vi "UpdateElement(Single).vi"(7 "Qualified Name":string, 8 "error in (no error)":errorcluster, 9 "Value":string, 10 "Key":string, 11 "ConfigManager.Text in":refnum<class "ConfigManager.Text.lvclass">) -> (0 "error out":errorcluster, 3 "ConfigManager.Text out":refnum<class "ConfigManager.Text.lvclass">)   [LabVIEW 2013, in "CfgManager.Text.lvlib" / "ConfigManager.Text.lvclass"]
uses:
  ConfigManager.Text.lvclass
  ConfigManager.Text.lvclass/ConfigManager.Text.ctl
  Update -- cluster.ctl
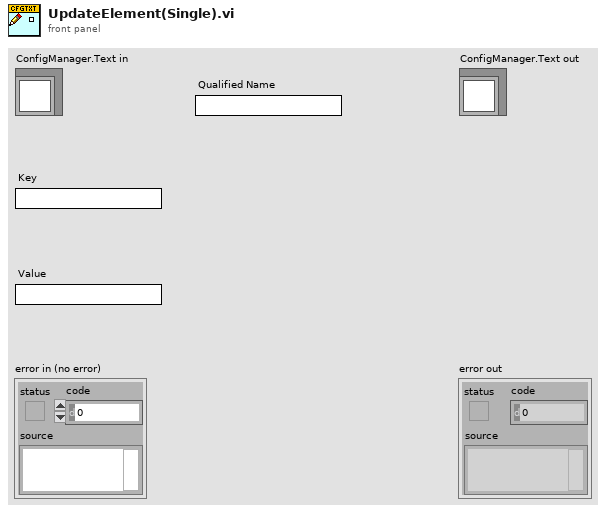
[diagram p1: front panel]
types:
  T1 = typedef "CfgManager.Text.lvlib/ConfigManager.Text.lvclass/Update -- cluster.ctl" = cluster{"Qualified Name":string[], "Keys":string[], "Values":string[]}
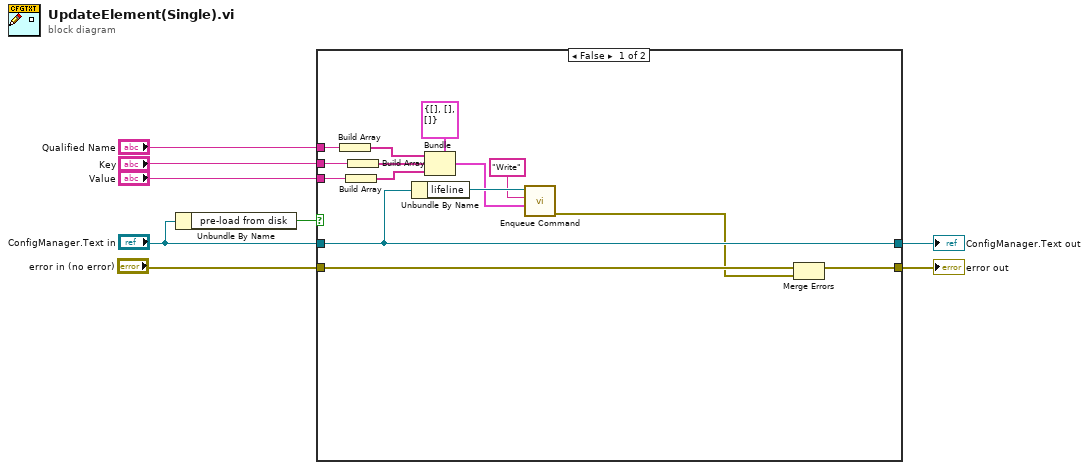
[diagram p0: block diagram]
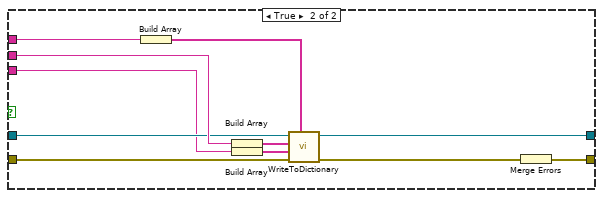
[diagram p2: hidden frame]
diagram:
  n1 = Unbundle By Name("ConfigManager.Text in") -> ("pre-load from disk"=w8:bool)
  n2 = case shown="False" w8 {
    tunnel: [w20 w33] -> w5
    tunnel: [w15 w29] -> w6
    tunnel: "Qualified Name" -> [w22 w30]
    tunnel: "error in (no error)" -> [w21 w24]
    tunnel: "Key" -> [w13 w32]
    tunnel: "ConfigManager.Text in" -> [w15 w31]
    tunnel: "Value" -> [w12 w25]
    frame False {
      n3 = Build Array(w22) -> (w9:string[])
      n4 = Build Array(w12) -> (w10:string[])
      n5 = Build Array(w13) -> (w19:string[])
      n6 = Unbundle By Name(w15) -> ("lifeline"=w18:refnum<queue>)
      n7 = Bundle(cluster=T1 {"Qualified Name"=[], "Keys"=[], "Values"=[]} ("Update"), "Qualified Name"=w9, "Keys"=w19, "Values"=w10) -> (w16:T1)
      n8 = call "Enqueue Command.vi"("args"=w16, "command"="Write", "Queue in"=w18) -> ("error out"=w14:errorcluster)  [unwired: 7 in, 1 out]
      n9 = Merge Errors(w21, w14) -> (w20:errorcluster)
    }
    frame True {
      n10 = Build Array(w30) -> (w23:string[])
      n11 = Build Array(w32) -> (w27:string[])
      n12 = Build Array(w25) -> (w26:string[])
      n13 = call "WriteToDictionary.vi"("Qualified Name"=w23, "error in (no error)"=w24, "Values"=w26, "Keys"=w27, "ConfigManager.Text in"=w31) -> ("error out"=w28:errorcluster, "ConfigManager.Text out"=w29:refnum<class "ConfigManager.Text.lvclass">)  [unwired: 5 in]
      n14 = Merge Errors(w28) -> (w33:errorcluster)
    }
  }
  "error out" <- w5
  "ConfigManager.Text out" <- w6
